vi "labview2tikz_WaveformGraph_WaveformData.vi"(8 "error in (no error)":errorcluster, 10 "file (use dialog)":path, 11 "WaveformGraph in":refnum<vi>) -> (0 "error out":errorcluster, 3 "result string":string)   [LabVIEW 2012]
uses:
  pgfPlotPlot_tdef.ctl
  <vilib>/Waveform/WDTOps.llb/WDT Get Waveform Time Array DBL.vi
  pgfPlotAxis_tdef.ctl
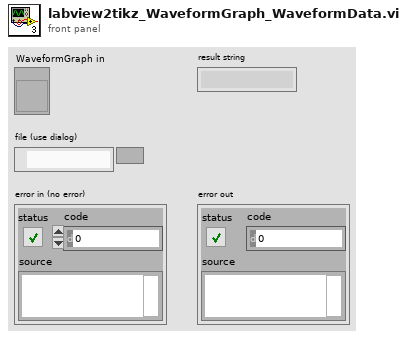
[diagram p1: front panel]
types:
  T1 = typedef "pgfPlotAxis_tdef.ctl" = cluster{"xmin":dbl, "xmax":dbl, "ymin":dbl, "ymax":dbl, "xLabel":string, "yLabel":string}
  T2 = typedef "pgfPlotPlot_tdef.ctl" = cluster{"LineStyle":u8, "LineWidth":u8, "PlotColor":u32, "Marker":u8, "PlotName":string, "x values":dbl[], "y values":dbl[]}
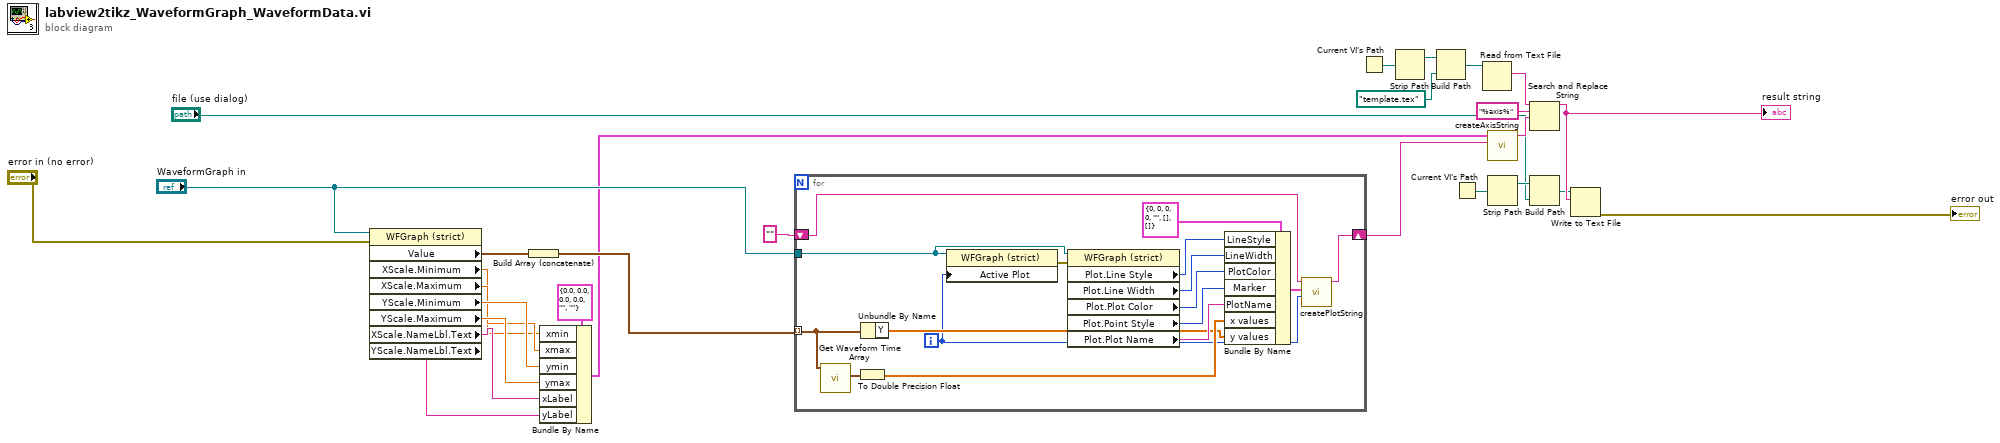
[diagram p0: block diagram]
diagram:
  n1 = property class="WFGraph (strict)"(reference="WaveformGraph in", error in="error in (no error)") -> ("Value"=w9:waveform(dbl)[], "XScale.Minimum"=w13:dbl, "XScale.Maximum"=w14:dbl, "YScale.Minimum"=w15:dbl, "YScale.Maximum"=w16:dbl, "XScale.NameLbl.Text"=w17:string, "YScale.NameLbl.Text"=w18:string)  [unwired: 2 out]
  n2 = Build Array (concatenate)(w9) -> (w27:waveform(dbl)[])
  n3 = Bundle By Name(cluster=T1 {"xmin"=0.0, "xmax"=0.0, "ymin"=0.0, "ymax"=0.0, "xLabel"="", "yLabel"=""} ("Input"), "xmin"=w13, "xmax"=w14, "ymin"=w15, "ymax"=w16, "xLabel"=w17, "yLabel"=w18) -> (w19:T1)
  n4 = for {
    tunnel: "WaveformGraph in" -> [w43]
    tunnel: w27 -> [w40] mode=indexing
    shift-right: [w39] -> w22
    shift-left: "" -> [w29]
    i -> [w28]
    n5 = call-poly <vilib>:"Get Waveform Time Array.vi"("waveform in"=w40) -> ("X array"=w42:timestamp[])  [unwired: 9 in, 1 out]
    n6 = To Double Precision Float(number=w42) -> (double precision float=w31:dbl[])
    n7 = Unbundle By Name(w40) -> ("Y"=w30:dbl[])
    n8 = property class="WFGraph (strict)"(reference=w43, "Active Plot"=w28) -> (error out=w41:errorcluster)  [unwired: 1 in, 1 out]
    n9 = property class="WFGraph (strict)"(reference=w43, error in=w41) -> ("Plot.Line Style"=w37:u8, "Plot.Line Width"=w36:u8, "Plot.Plot Color"=w32:u32, "Plot.Point Style"=w35:u8, "Plot.Plot Name"=w34:string)  [unwired: 2 out]
    n10 = Bundle By Name(cluster=T2 {"LineStyle"=0, "LineWidth"=0, "PlotColor"=0, "Marker"=0, "PlotName"="", "x values"=[], "y values"=[]}, "LineStyle"=w37, "LineWidth"=w36, "PlotColor"=w32, "Marker"=w35, "PlotName"=w34, "x values"=w31, "y values"=w30) -> (w33:T2)
    n11 = call "createPlotString.vi"("current plot number"=w28, "Plot Data"=w33, "plot string in"=w29) -> ("plot string out"=w39:string)  [unwired: 8 in]
  }
  n12 = Current VI's Path() -> (path=w1:path)
  n13 = Strip Path(path=w1) -> (stripped path=w2:path)  [unwired: 1 out]
  n14 = Build Path(base path=w2, name or relative path=path "template.tex" ("file (use dialog)")) -> (appended path=w4:path)
  n15 = Current VI's Path() -> (path=w7:path)
  n16 = Read from Text File(file (use dialog)=w4) -> (text=w11:string)  [unwired: 3 in, 3 out]
  n17 = call "createAxisString.vi"("PlotsString"=w22, "Input Data"=w19) -> ("AxisString"=w21:string)  [unwired: 9 in]
  n18 = Strip Path(path=w7) -> (stripped path=w6:path)  [unwired: 1 out]
  n19 = Search and Replace String(input string=w11, search string="%axis%", replace string=w21) -> (result string=w23:string)  [unwired: 5 in, 3 out]
  "result string" <- w23
  n20 = Build Path(base path=w6, name or relative path="file (use dialog)") -> (appended path=w8:path)
  n21 = Write to Text File(file (use dialog)=w8, text=w23) -> (error out=→"error out":errorcluster)  [unwired: 2 in, 2 out]
